vi "U2000_USB_PM_Fetch Measurement.vi"(8 "error in (no error)":errorcluster, 10 "Timeout (10000 ms)":u32=10000, 11 "VISA resource name":refnum<visa-resource-name>) -> (0 "error out":errorcluster, 2 "Measurement":dbl, 3 "VISA resource name out":refnum<visa-resource-name>)   [LabVIEW 2014]
doc: "Queries and retrieves measurement results.\n\nNote: \nUse this VI only with other low-level VIs. The high-level VIs automatically incorporate this functionality. This VI does not check the instrument status."
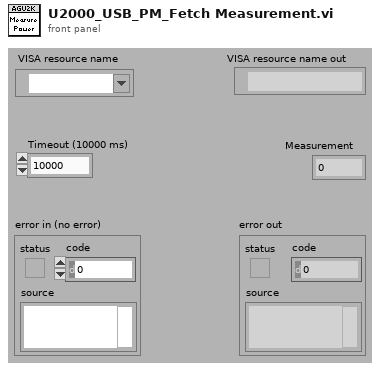
[diagram p1: front panel]
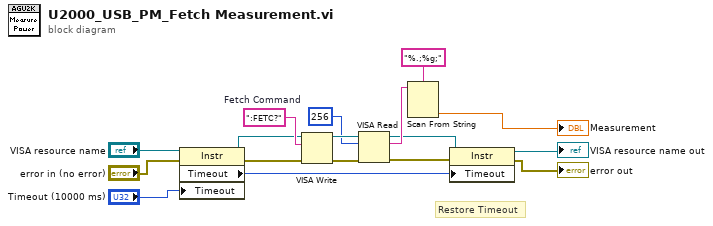
[diagram p0: block diagram]
diagram:
  w17 = ":FETC?"  # Fetch Command
  # "Restore Timeout"
  n1 = property class="Instr"(reference="VISA resource name", error in="error in (no error)", "Timeout"="Timeout (10000 ms)") -> (reference out=w1:refnum<visa-resource-name>, error out=w2:errorcluster, "Timeout"=w3:u32)
  n2 = VISA Write(VISA resource name=w1, write buffer=w17, error in (no error)=w2) -> (VISA resource name out=w16:refnum<visa-resource-name>, error out=w15:errorcluster)  [unwired: 1 out]
  n3 = VISA Read(VISA resource name=w16, byte count=u32 256, error in (no error)=w15) -> (VISA resource name out=w7:refnum<visa-resource-name>, read buffer=w11:string, error out=w6:errorcluster)  [unwired: 1 out]
  n4 = Scan From String(format string="%.;%g;", input string=w11) -> (output 1=→"Measurement":dbl)  [unwired: 2 in, 4 out]
  n5 = property class="Instr"(reference=w7, error in=w6, "Timeout"=w3) -> (reference out=→"VISA resource name out":refnum<visa-resource-name>, error out=→"error out":errorcluster)
